vi "Untitled 1.vi"() -> ()   [LabVIEW 2015]
panel:
  out "Array":cluster{"Vel":dbl, dbl, dbl, dbl}[](array[cluster])
  in  "Array 2":T1(array[cluster])
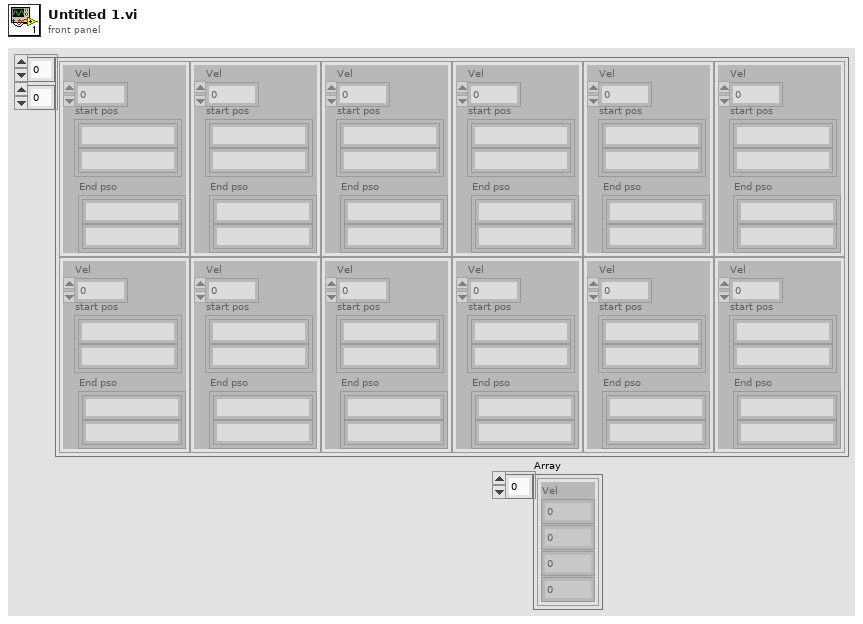
[diagram p1: front panel]
types:
  T1 = cluster{"Vel":dbl, "start pos":cluster{string, string}, "End pso":cluster{string, string}}[][]
  T2 = cluster{"Vel":dbl, "start pos":cluster{string, string}, "End pso":cluster{string, string}}[]
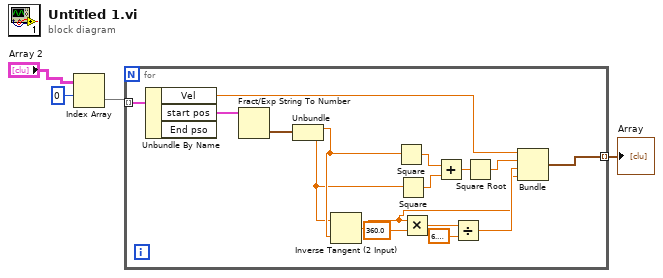
[diagram p0: block diagram]
diagram:
  n1 = Index Array(array="Array 2", index (row)=0) -> (element=w2:T2)  [unwired: 1 in]
  n2 = for {
    tunnel: w2 -> [w20] mode=indexing
    tunnel: [w12] -> w1 mode=indexing
    n3 = Unbundle By Name(w20) -> ("Vel"=w13:dbl, "start pos"=w19:cluster{string, string})  [unwired: 1 out]
    n4 = Fract/Exp String To Number(string=w19) -> (number=w18:cluster{dbl, dbl})  [unwired: 3 in, 1 out]
    n5 = Unbundle(w18) -> (w11:dbl, w10:dbl)
    n6 = Inverse Tangent (2 Input)(1:w11, 2:w10) -> (0:w5:dbl)
    n7 = Square(x=w11) -> (x^2=w17:dbl)
    n8 = Square(x=w10) -> (x^2=w16:dbl)
    n9 = Multiply(x=w5, y=360.0) -> (x*y=w8:dbl)
    n10 = Add(x=w17, y=w16) -> (x+y=w15:dbl)
    n11 = Divide(x=w8, y=6.283185307179586) -> (x/y=w6:dbl)
    n12 = Square Root(x=w15) -> (sqrt(x)=w14:dbl)
    n13 = Bundle("Vel"=w13, w14, w6, w5) -> (w12:cluster{"Vel":dbl, dbl, dbl, dbl})  [unwired: 1 in]
  }
  "Array" <- w1
